vi "写测量文件.vi"() -> ()   [LabVIEW 2010]
uses:
  Instance           1 18Saved   写测量文件 .vi
  Instance           2 18Saved   写测量文件 .vi
panel:
  in  "File Name":path=path "test.lvm" caption="文件名"
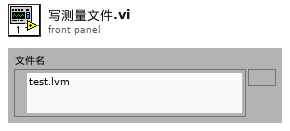
[diagram p1: front panel]
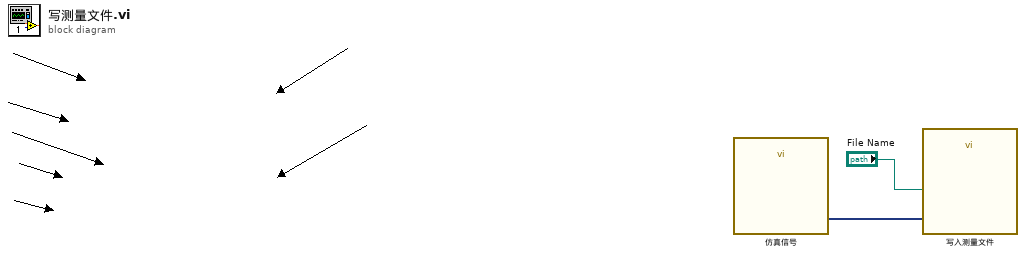
[diagram p0: block diagram]
diagram:
  n1 = call "仿真信号"() -> ("正弦"=w2:dynamicdata)  [unwired: 14 in, 1 out]
  n2 = call "写入测量文件"("Signals"=w2, "File Name"="File Name") -> ()  [unwired: 15 in, 3 out]
